vi "Boolean Latch.vi"(1 "Input":bool) -> (21 "Output":bool)   [LabVIEW 2019, in "G3 library.lvlib"]
uses:
  G3 library.lvlib
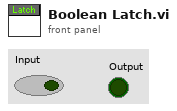
[diagram p1: front panel]
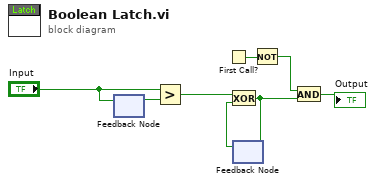
[diagram p0: block diagram]
diagram:
  n1 = feedback #1() -> (w6:bool)  [unwired: 1 in]
  n2 = feedback-in #1("Input") -> ()
  n3 = Greater?(x="Input", y=w6) -> (0:w7:bool)
  n4 = First Call?() -> (First Call?: T/F=w2:bool)
  n5 = feedback #2() -> (w8:bool)  [unwired: 1 in]
  n6 = Exclusive Or(1:w8, 2:w7) -> (0:w3:bool)
  n7 = feedback-in #2(w3) -> ()
  n8 = Not(x=w2) -> (.not. x?=w1:bool)
  n9 = And(x=w1, y=w3) -> (x .and. y?=→"Output":bool)
